vi "ToTable.vi"(8 "error in":errorcluster, 9 "Table Index (0)":i32, 10 "variant":variant, 11 "Increment editor node in":refnum<class "Increment editor node.lvclass">) -> (0 "error out":errorcluster, 1 "row headers":string[](array[string]), 2 "table":string[][](array[string]), 3 "Increment editor node out":refnum<class "Increment editor node.lvclass">)   [LabVIEW 2015, in "Increment editor node.lvclass"]
doc: "Generates the strings needed to display on a table based on the information found in the engine and module configuration classes."
uses:
  Increment editor node.lvclass
  module/configuration/Increment configuration.lvclass
  <vilib>/NI/Module Execution Interface/Engine Configuration/engine configuration.lvclass
  module/configuration/Increment configuration.lvclass/Increment configuration.ctl
  <vilib>/NI/Configuration Framework/serializable configuration/NISE_CEF_serializable configuration.lvclass/NISE_CEF_serializable configuration.ctl
  <vilib>/NI/Tag Bus/tag/tag descriptor.lvclass/tag descriptor.ctl
  module/configuration/Read Lines.vi
  <vilib>/Utility/LVClass/Get LV Class Name.vi
  <vilib>/NI/Configuration Framework/error generator/NISE_error generator.vi
  <vilib>/NI/Tag Bus Module Framework/channel/TBM channel.lvclass
  <vilib>/NI/Tag Bus/tag/tag descriptor.lvclass
  <vilib>/NI/Configuration Framework/serializable configuration/NISE_CEF_serializable configuration.lvclass
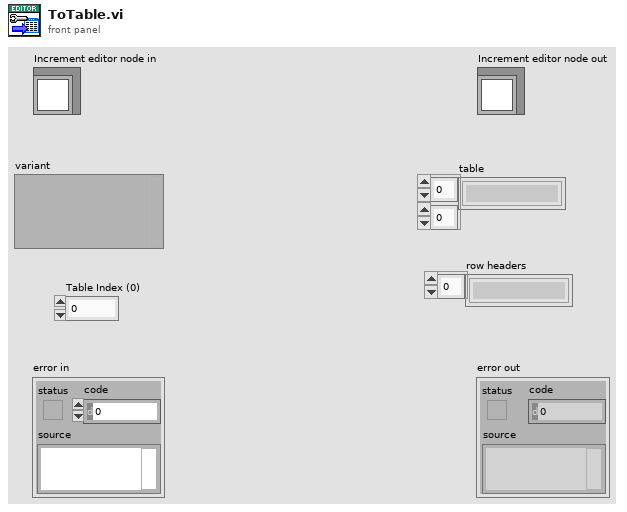
[diagram p1: front panel]
types:
  T1 = typedef "Increment configuration.lvclass/Line.ctl" = cluster{"Name":string, "channel in":refnum<class "TBM channel.lvclass">, "channel out":refnum<class "TBM channel.lvclass">}
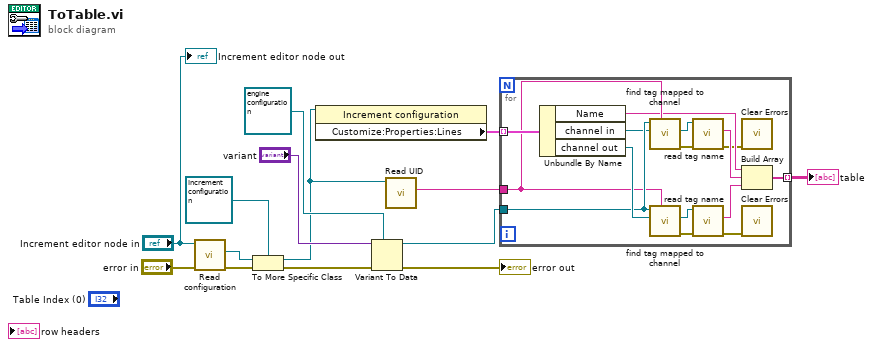
[diagram p0: block diagram]
diagram:
  n1 = call-dynamic "Read configuration.vi"("error in"="error in", "Increment editor node in"="Increment editor node in") -> ("error out"=w14:errorcluster, "configuration"=w5:refnum<class "NISE_CEF_serializable configuration.lvclass">)  [unwired: 7 in, 1 out]
  n2 = To More Specific Class(target class=refnum<class "Increment configuration.lvclass"> refnum ("tag bus configurable plugin module configuration"), reference=w5, error in=w14) -> (specific class reference=w4:refnum<class "Increment configuration.lvclass">, error out=w2:errorcluster)
  n3 = property class="Increment configuration"(reference=w4) -> ("Customize:Properties:Lines"=w11:T1[])  [unwired: 1 in, 2 out]
  n4 = Variant To Data(error in=w2, type=refnum<class "engine configuration.lvclass"> refnum ("engine configuration"), Variant="variant") -> (data=w8:refnum<class "engine configuration.lvclass">, error out=→"error out":errorcluster)
  n5 = call <vilib>:"Read UID.vi"("configuration in"=w4) -> ("instance id"=w3:string)  [unwired: 8 in, 2 out]
  n6 = for {
    tunnel: w11 -> [w29] mode=indexing
    tunnel: w8 -> [w24]
    tunnel: [w25] -> w6 mode=indexing
    tunnel: w3 -> [w23]
    n7 = Unbundle By Name(w29) -> ("Name"=w20:string, "channel in"=w15:refnum<class "TBM channel.lvclass">, "channel out"=w26:refnum<class "TBM channel.lvclass">)
    n8 = call <vilib>:"find tag mapped to channel.vi"("owner"=w23, "channel"=w15, "engine configuration in"=w24) -> ("error out"=w18:errorcluster, "tag"=w22:refnum<class "tag descriptor.lvclass">)  [unwired: 6 in, 1 out]
    n9 = call <vilib>:"find tag mapped to channel.vi"("owner"=w23, "channel"=w26, "engine configuration in"=w24) -> ("error out"=w19:errorcluster, "tag"=w28:refnum<class "tag descriptor.lvclass">)  [unwired: 6 in, 1 out]
    n10 = call <vilib>:"read tag name.vi"("error in"=w18, "system tag in"=w22) -> ("error out"=w17:errorcluster, "name"=w21:string)  [unwired: 7 in, 1 out]
    n11 = call <vilib>:"read tag name.vi"("error in"=w19, "system tag in"=w28) -> ("error out"=w16:errorcluster, "name"=w27:string)  [unwired: 7 in, 1 out]
    n12 = call <vilib>:"Clear Errors.vi"("error in (no error)"=w17) -> ()  [unwired: 5 in, 2 out]
    n13 = Build Array(w20, w21, w27) -> (w25:string[])
    n14 = call <vilib>:"Clear Errors.vi"("error in (no error)"=w16) -> ()  [unwired: 5 in, 2 out]
  }
  "table" <- w6
  "Increment editor node out" <- "Increment editor node in"
